vi "set_thermocouple_calibration_single_point.vi"(8 "error in (no error)":errorcluster, 10 "Offset (deg C)":dbl, 11 "VISA Refnum in":refnum<visa-resource-name>) -> (0 "error out":errorcluster, 3 "VISA Refnum out":refnum<visa-resource-name>)   [LabVIEW 2018]
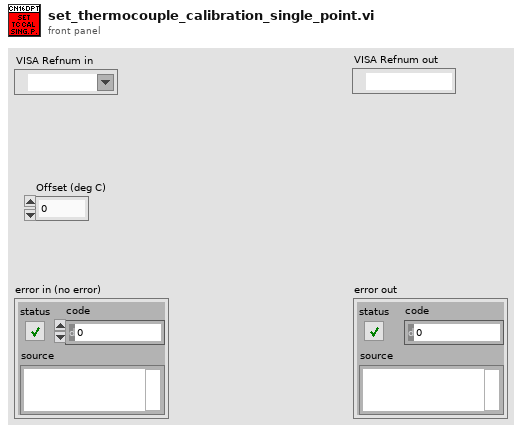
[diagram p1: front panel]
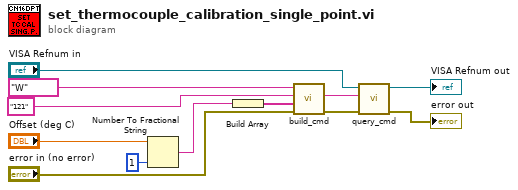
[diagram p0: block diagram]
diagram:
  n1 = Number To Fractional String(number="Offset (deg C)", precision (6)=i16 1) -> (F-format string=w2:string)  [unwired: 2 in]
  n2 = Build Array(w2) -> (w4:string[])
  n3 = call "build_cmd.vi"("error in (no error)"="error in (no error)", "Parameter list"=w4, "Command ID"="121", "Command class"="W") -> ("error out"=w7:errorcluster, "Command"=w6:string)  [unwired: 6 in]
  n4 = call "query_cmd.vi"("error in (no error)"=w7, "Command"=w6, "VISA resource name"="VISA Refnum in") -> ("error out"=→"error out":errorcluster, "VISA resource name out"=→"VISA Refnum out":refnum<visa-resource-name>)  [unwired: 6 in, 1 out]
